vi "IsBaseInRange.vi"(0 "SetValueInfo":refnum<vi>[](array[refnum]), 2 "DIMControSet":refnum<vi>[](array[refnum]), 3 "ListOfBases_Data":refnum<vi>, 5 "NewVal in":dbl, 8 "Base Name":string) -> (16 "NewVal Out":dbl, 19 "In Range":bool)   [LabVIEW 2014, in "Panels.lvlib"]
uses:
  Panels.lvlib
  Instance           1 21Saved   IsBaseInRange .vi
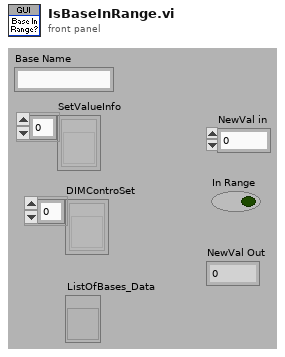
[diagram p1: front panel]
types:
  T1 = cluster{"data":string, "no link":bool, "quality":i32, "timeStamp":dbl}
  T2 = cluster{"data":dbl[], "no link":bool, "quality":i32, "timeStamp":dbl}
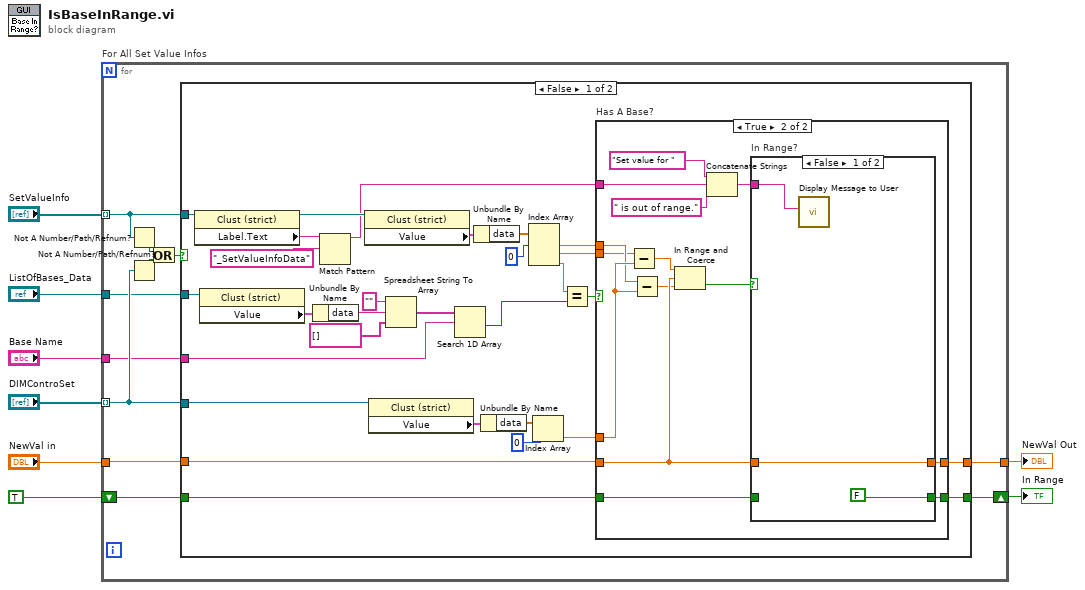
[diagram p0: block diagram]
diagram:
  n1 = for "For All Set Value Infos" {
    tunnel: "SetValueInfo" -> [w15] mode=indexing
    tunnel: "DIMControSet" -> [w14] mode=indexing
    tunnel: "NewVal in" -> [w19]
    tunnel: [w18] -> w8
    shift-right: [w17] -> w5
    shift-left: TRUE -> [w16]
    tunnel: "ListOfBases_Data" -> [w10]
    tunnel: "Base Name" -> [w9]
    n2 = Not A Number/Path/Refnum?(number/path/refnum=w15) -> (NaN/Path/Refnum?=w12:bool)
    n3 = Not A Number/Path/Refnum?(number/path/refnum=w14) -> (NaN/Path/Refnum?=w11:bool)
    n4 = Or(x=w12, y=w11) -> (x .or. y?=w13:bool)
    n5 = case shown="False" w13 {
      tunnel: w19 -> [w48 w70]
      tunnel: [w47 w70] -> w18
      tunnel: [w46 w71] -> w17
      tunnel: w14 -> [w45 _]
      tunnel: w16 -> [w44 w71]
      tunnel: w15 -> [w32 _]
      tunnel: w10 -> [w30 _]
      tunnel: w9 -> [w20 _]
      frame False {
        n6 = property class="Clust (strict)"(reference=w32) -> (reference out=w31:refnum<vi>, "Label.Text"=w33:string)  [unwired: 1 in, 1 out]
        n7 = property class="Clust (strict)"(reference=w30) -> ("Value"=w29:T1)  [unwired: 1 in, 2 out]
        n8 = Unbundle By Name(w29) -> ("data"=w28:string)
        n9 = Match Pattern(string=w33, regular expression="_SetValueInfoData") -> (before substring=w24:string)  [unwired: 1 in, 3 out]
        n10 = property class="Clust (strict)"(reference=w31) -> ("Value"=w35:T2)  [unwired: 1 in, 2 out]
        n11 = property class="Clust (strict)"(reference=w45) -> ("Value"=w34:T2)  [unwired: 1 in, 2 out]
        n12 = Spreadsheet String To Array(format string="", spreadsheet string=w28, array type (2D Dbl)=string[] []) -> (array=w25:string[])  [unwired: 1 in]
        n13 = Search 1D Array(1D array=w25, element=w20) -> (index of element=w22:i32)  [unwired: 1 in]
        n14 = Unbundle By Name(w35) -> ("data"=w42:dbl[])
        n15 = Unbundle By Name(w34) -> ("data"=w38:dbl[])
        n16 = Index Array(array=w42, index #1=0 ("index")) -> (element #1=w40:dbl, element #2=w39:dbl, element #3=w23:dbl)  [unwired: 2 in]
        n17 = Index Array(array=w38, index=0) -> (element=w36:dbl)
        n18 = Equal?(x=w23, y=w22) -> (x = y?=w21:bool)
        n19 = case "Has A Base?" shown="True" w21 {
          tunnel: w40 -> [_ w53]
          tunnel: w39 -> [_ w52]
          tunnel: w48 -> [w49 w59]
          tunnel: w36 -> [_ w64]
          tunnel: w44 -> [w50 w61]
          tunnel: [w50 w60] -> w46
          tunnel: [w49 w58] -> w47
          tunnel: w24 -> [_ w55]
          frame False {
          }
          frame True {
            n20 = Subtract(x=w52, y=w64) -> (x-y=w63:dbl)
            n21 = Subtract(x=w53, y=w64) -> (x-y=w51:dbl)
            n22 = In Range and Coerce(upper limit=w63, x=w59, lower limit=w51) -> (In Range?=w62:bool)  [unwired: 1 out]
            n23 = Concatenate Strings("Set value for " ("string"), w55, " is out of range." ("string")) -> (w54:string)
            n24 = case "In Range?" shown="False" w62 {
              tunnel: w61 -> [_ w69]
              tunnel: [FALSE w69] -> w60
              tunnel: [w66 w68] -> w58
              tunnel: w59 -> [w66 w68]
              tunnel: w54 -> [w65 _]
              frame False {
                n25 = call "Display Message to User"("Message"=w65) -> ()  [unwired: 9 in, 2 out]
              }
              frame True {
              }
            }
          }
        }
      }
      frame True {
      }
    }
  }
  "In Range" <- w5
  "NewVal Out" <- w8
